vi "Filter Zeros (fast).vi"(11 "Array in":dbl[](array[numeric])) -> (3 "Array out":dbl[](array[numeric]))   [LabVIEW 2018, in "Video Processor.lvclass"]
doc: "Filters zeros from the array, but does not maintain the original order of the elements in order to save time."
uses:
  Video Processor.lvclass
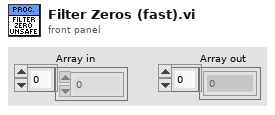
[diagram p1: front panel]
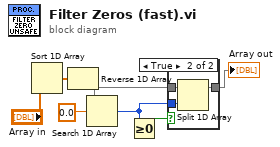
[diagram p0: block diagram]
diagram:
  n1 = Sort 1D Array(array="Array in") -> (sorted array=w5:dbl[])
  n2 = Reverse 1D Array(array=w5) -> (reversed array=w6:dbl[])
  n3 = Search 1D Array(1D array=w6, element=0.0 ("Element")) -> (index of element=w2:i32)  [unwired: 1 in]
  n4 = Greater Or Equal To 0?(x=w2) -> (x >= 0?=w1:bool)
  n5 = case shown="True" w1 {
    tunnel: w6 -> [w8 w11]
    tunnel: w2 -> [_ w10]
    tunnel: [w8 w9] -> w7
    frame False {
    }
    frame True {
      n6 = Split 1D Array(array=w11, index=w10) -> (first subarray=w9:dbl[])  [unwired: 1 out]
    }
  }
  "Array out" <- w7
